vi "PH_ImageCoG_Plotter.Show Image.vi"(0 "i ref in":refnum<vi>, 5 "error in":errorcluster) -> (14 "i ref out":refnum<vi>, 19 "error out":errorcluster)   [LabVIEW 2014, in "PH_ImageCoG_Plotter.lvlib"]
doc: "This VI sets a copy of the image, sets additional information and plots it at the GUI element."
uses:
  PH_ImageCoG_Plotter.lvlib
  PH_Basics/PH_Image_Common/PH_Image_Common.lvlib
  PH_Basics/PH_Img_BaseClass/PH_Img_BaseClass.lvlib
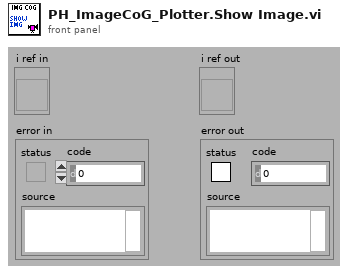
[diagram p1: front panel]
types:
  T1 = typedef "PH_ImageCoG_Plotter.lvlib/PH_ImageCoG_Plotter.i attribute.ctl" = cluster{"GUI Refs":cluster{"Delete":refnum<vi>, "Calibration status":refnum<vi>, "BI subtracted":refnum<vi>, "calc Beam Anal":refnum<vi>, "CoG - x":refnum<vi>, "CoG - y":refnum<vi>, "Type":refnum<vi>, "Center":refnum<vi>, "exp - X":refnum<vi>, "exp - Y":refnum<vi>, "Delta - X":refnum<vi>, "Delta - Y":refnum<vi>, "Available Cams":refnum<vi>, "CoG X":refnum<vi>, "CoG Y":refnum<vi>, "Delta X":refnum<vi>, "Delta Y":refnum<vi>, "Export Data":refnum<vi>, "Calibration data":refnum<vi>}, "Calibration":cluster{"Status":T2, "Calibration data":T3, "Calibration Data File":path}, "Beam Analysis":cluster{"on":bool, "exp - X":i32, "exp - Y":i32, "Type":bool, "Data":cluster{"current time":timestamp, "CoG-x":dbl, "CoG-y":dbl, "Delta-x":dbl, "Delta-y":dbl}[], "Datasets strored":i32, "Dataarray Size":i32}, "Cam instances":string[], "DIM Service Events":T4[], "Images":cluster{"Background":T7, "OP":T7, "GUI":T7}}
  T2 = typedef "PH_StatusHandler.lvlib/PH_StatusHandler.Status.ctl" = i16
  T3 = typedef "PH_ImageCalibrator.lvlib/PH_ImageCalibrator.Calibration Data.ctl" = cluster{"Date":string, "Time":string, "Cam Settings":cluster{"Cam ID":string, "Gain":dbl, "Brightness":dbl, "Shutter":dbl, "Cam Error":bool, "Mode":i32}, "Background Image":cluster{"Image":dbl[][], "Image Error":bool}, "Linear Calibration":cluster{"Calibration Factor":dbl, "not mm or mrad":bool}, "Energy Calibration":cluster{"Calibration Factor":dbl, "no mJ":bool}}
  T4 = typedef "BaseProcess.lvlib/BaseProcess.event definition.ctl" = cluster{"CAEEvtDef":T5, "Data Descriptor":T6}
  T5 = typedef "CAEObj.lvlib/CAEObj.event definition.ctl" = cluster{"URL":string, "enable":bool, "ignoreResID":bool}
  T6 = typedef "BaseProcess.lvlib/BaseProcess.descriptor string definition.ctl" = string
  T7 = typedef "IMAQ Image.ctl" = refnum<image>
  T8 = cluster{"current time":timestamp, "CoG-x":dbl, "CoG-y":dbl, "Delta-x":dbl, "Delta-y":dbl}[]
  T9 = cluster{"current time":timestamp, "CoG-x":dbl, "CoG-y":dbl, "Delta-x":dbl, "Delta-y":dbl}
  T10 = typedef "PH_Img_BaseClass.lvlib/PH_Img_BaseClass.i attribute.ctl" = cluster{"GUI Refs":T11, "Timeout Image [ms]":i32, "Default Periodic Period [ms]":i32, "Camera":cluster{"Instancename":string, "Notifier":refnum<notifier>}, "Palette":T12, "Cam Settings":cluster{"Cam ID":string, "Gain":dbl, "Brightness":dbl, "Shutter":dbl, "Cam Info Failure":bool, "Mode":i32}}
  T11 = typedef "PH_Img_BaseClass.lvlib/PH_Img_BaseClass.GUI Refs.ctl" = cluster{"Timeout":refnum<vi>, "Image":refnum<vi>, "Palette":refnum<vi>, "Timeout Set":refnum<vi>}
  T12 = typedef "PH_Img_BaseClass.lvlib/PH_Img_BaseClass.Palette.ctl" = i32
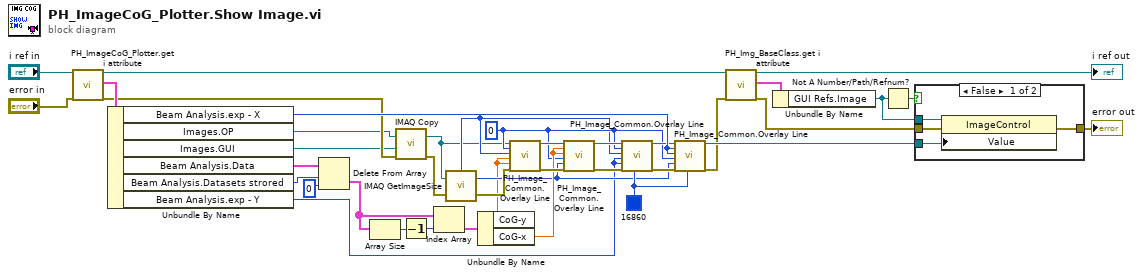
[diagram p0: block diagram]
diagram:
  w20 = 0 ("Start y")
  w30 = u32 16860 ("Color (red)")
  n1 = call "PH_ImageCoG_Plotter.get i attribute.vi"("i ref in"="i ref in", "error in (no error)"="error in") -> ("i ref out"=w9:refnum<vi>, "i attribute"=w38:T1, "error out"=w5:errorcluster)  [unwired: 15 in]
  n2 = Unbundle By Name(w38) -> ("Beam Analysis.exp - X"=w33:i32, "Images.OP"=w2:T7, "Images.GUI"=w1:T7, "Beam Analysis.Data"=w13:T8, "Beam Analysis.Datasets strored"=w11:i32, "Beam Analysis.exp - Y"=w14:i32)
  n3 = Delete From Array(array=w13, length=w11, index=0) -> (deleted portion=w12:T8)  [unwired: 1 out]
  n4 = Array Size(array=w12) -> (size(s)=w25:i32)
  n5 = call "IMAQ Copy"("error in (no error)"=w5, "Image Dst"=w1, "Image Src"=w2) -> ("error out"=w16:errorcluster, "Image Dst Out"=w15:T7)  [unwired: 3 in]
  n6 = Decrement(x=w25) -> (x-1=w26:i32)
  n7 = Index Array(array=w12, index=w26) -> (element=w24:T9)
  n8 = call "IMAQ GetImageSize"("Image"=w15, "error in (no error)"=w16) -> ("Y Resolution"=w18:i32, "X Resolution"=w19:i32, "error out"=w22:errorcluster)  [unwired: 2 in]
  n9 = Unbundle By Name(w24) -> ("CoG-y"=w17:dbl, "CoG-x"=w23:dbl)
  n10 = call "PH_Image_Common.Overlay Line.vi"("Image"=w15, "Start x"=w20, "End x"=w19, "Start y"=w17, "End y"=w17, "error in (no error)"=w22) -> ("Image Out"=w28:T7, "error out"=w29:errorcluster)  [unwired: 12 in]
  n11 = call "PH_Image_Common.Overlay Line.vi"("Image"=w28, "Start x"=w23, "End x"=w23, "Start y"=w20, "End y"=w18, "error in (no error)"=w29) -> ("Image Out"=w27:T7, "error out"=w21:errorcluster)  [unwired: 12 in]
  n12 = call "PH_Image_Common.Overlay Line.vi"("Image"=w27, "Start x"=w20, "End x"=w19, "Start y"=w14, "End y"=w14, "error in (no error)"=w21, "Color (red)"=w30) -> ("Image Out"=w32:T7, "error out"=w31:errorcluster)  [unwired: 11 in]
  n13 = call "PH_Image_Common.Overlay Line.vi"("Image"=w32, "Start x"=w33, "End x"=w33, "Start y"=w20, "End y"=w18, "error in (no error)"=w31, "Color (red)"=w30) -> ("Image Out"=w34:T7, "error out"=w4:errorcluster)  [unwired: 11 in]
  n14 = call "PH_Img_BaseClass.get i attribute.vi"("i ref in"=w9, "error in (no error)"=w4) -> ("i ref out"=→"i ref out":refnum<vi>, "i attribute"=w7:T10, "error out"=w3:errorcluster)  [unwired: 15 in]
  n15 = Unbundle By Name(w7) -> ("GUI Refs.Image"=w6:refnum<vi>)
  n16 = Not A Number/Path/Refnum?(number/path/refnum=w6) -> (NaN/Path/Refnum?=w35:bool)
  n17 = case shown="False" w35 {
    tunnel: w6 -> [w41 _]
    tunnel: [w43 w44] -> w36
    tunnel: w34 -> [w40 _]
    tunnel: w3 -> [w42 w44]
    frame False {
      n18 = property class="ImageControl"(reference=w41, error in=w42, "Value"=w40) -> (error out=w43:errorcluster)  [unwired: 1 out]
    }
    frame True {
    }
  }
  "error out" <- w36
